vi "Translator.vi"(0 "Input":variant=variant("Function Name"=variant(string "Strip Path"), "Input Datatypes"=variant(string[] ["error", "int"]), "Inputs"=variant(string[] ["error in", "x"]), "Node refnum"=variant(refnum<vi> refnum), "Output Datatypes"=variant(string[] ["int"]), "Outputs"=variant(string[] ["a"])), 11 "error in (no error)":errorcluster) -> (4 "Output":variant=variant("Defines"=variant(string[] []), "Includes"=variant(string[] []), "Replaced Code"=variant(string "/* LabVIEW system function 'Strip Path' not found. */")), 15 "error out":errorcluster)   [LabVIEW 2014, in "LabVIEW Universal Trasncriptor Servo.lvlib"]
doc: "An example of how to create the Translator to convert the LabVIEW VIs to Arduino C code."
uses:
  LabVIEW Universal Trasncriptor Servo.lvlib
panel:
  out "Outputs":string[](array[string])
  out "Inputs":string[](array[string])
  out "Output Datatypes":string[](array[string])
  out "Input Datatypes":string[](array[string])
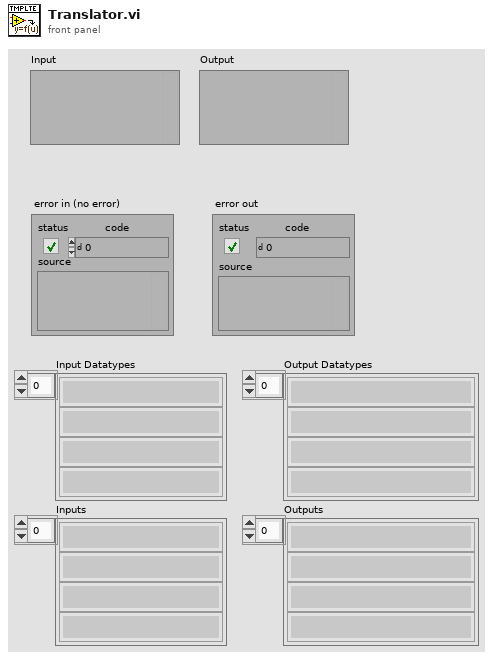
[diagram p1: front panel]
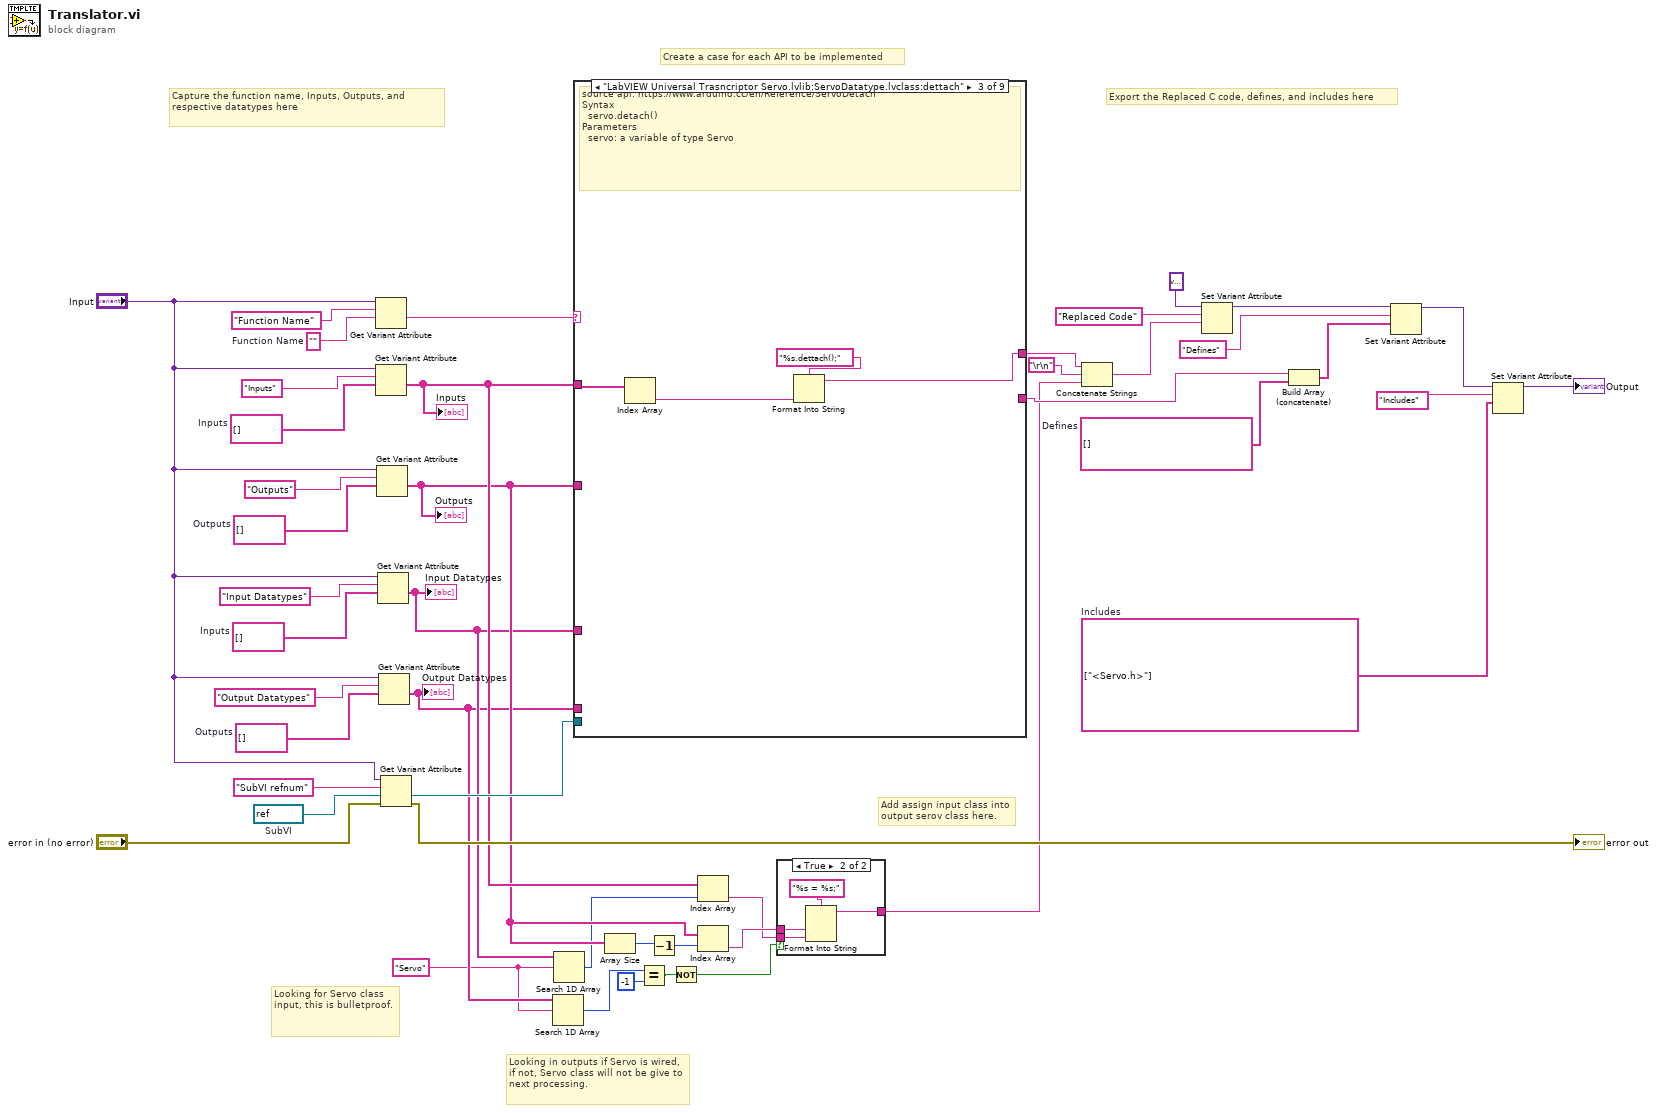
[diagram p0: block diagram]
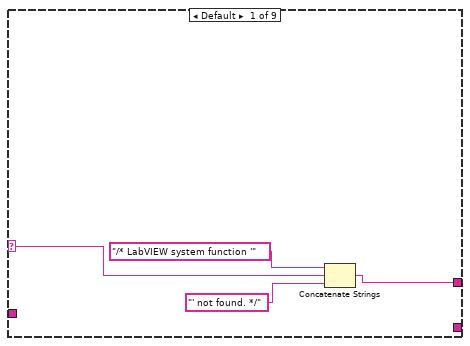
[diagram p3: hidden frame]
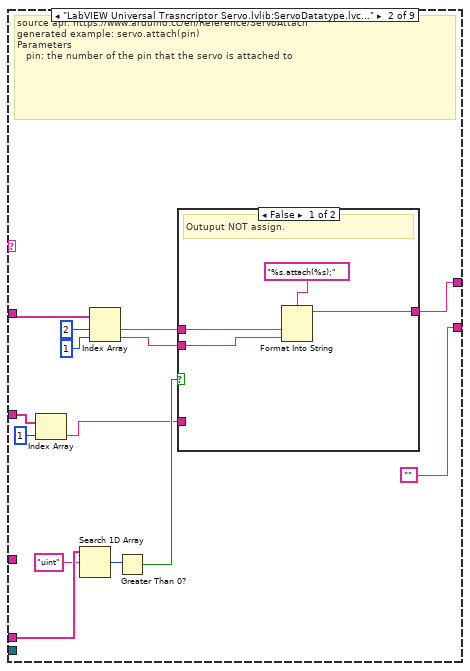
[diagram p4: hidden frame]
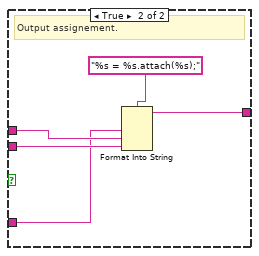
[diagram p5: hidden frame]
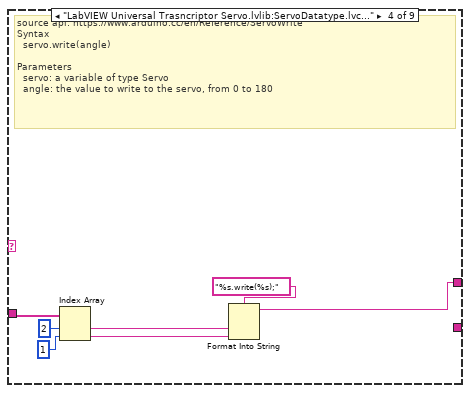
[diagram p6: hidden frame]
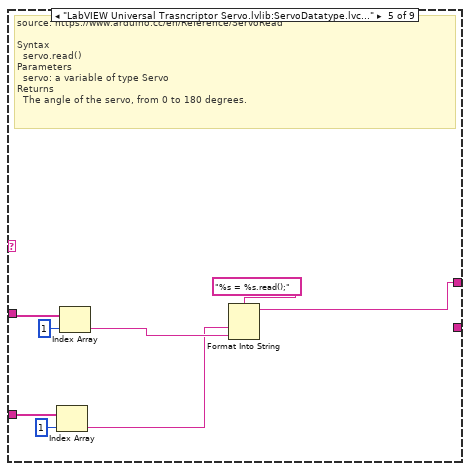
[diagram p7: hidden frame]
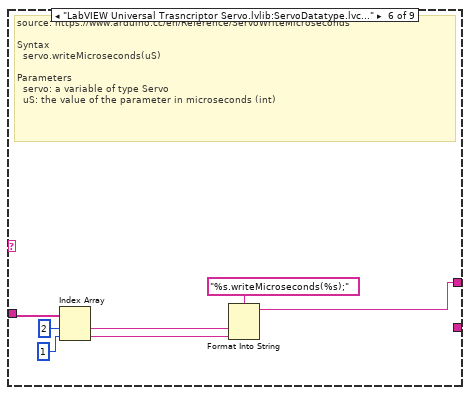
[diagram p8: hidden frame]
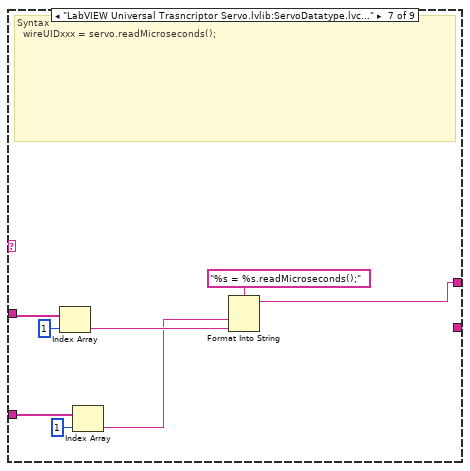
[diagram p9: hidden frame]
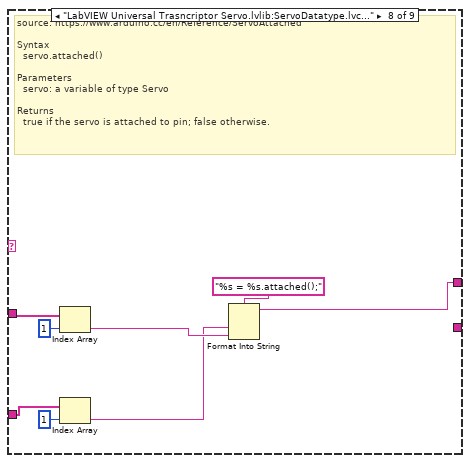
[diagram p10: hidden frame]
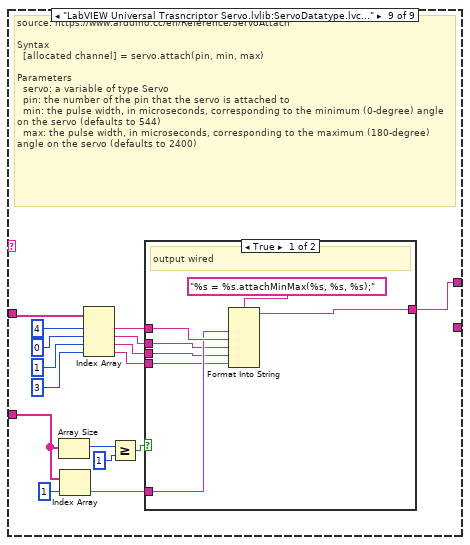
[diagram p11: hidden frame]
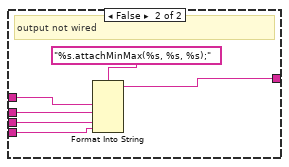
[diagram p12: hidden frame]
diagram:
  w2 = "Servo" ("format string")
  w26 = refnum<vi> refnum  # SubVI
  w21 = string[] []  # Defines
  w33 = string[] []  # Outputs
  w34 = string[] []  # Inputs
  w24 = string[] ["<Servo.h>"]  # Includes
  w42 = string[] []  # Outputs
  w43 = string[] []  # Inputs
  w44 = ""  # Function Name
  # "Looking for Servo class input, this is bulletproof."
  # "Looking in outputs if Servo is wired, if not, Servo class will not be give to next processing."
  # "Add assign input class into output serov class here."
  # "Capture the function name, Inputs, Outputs, and respective datatypes here"
  # "Export the Replaced C code, defines, and includes here"
  # "Create a case for each API to be implemented"
  n1 = Get Variant Attribute(Variant="Input", name="Function Name", default value (empty Variant)=w44) -> (value=w39:string)  [unwired: 1 in, 3 out]
  n2 = Get Variant Attribute(Variant="Input", name="Inputs", default value (empty Variant)=w43) -> (value=w10:string[])  [unwired: 1 in, 3 out]
  "Inputs" <- w10
  n3 = Get Variant Attribute(Variant="Input", name="Outputs", default value (empty Variant)=w42) -> (value=w9:string[])  [unwired: 1 in, 3 out]
  "Outputs" <- w9
  n4 = Get Variant Attribute(Variant="Input", name="Input Datatypes", default value (empty Variant)=w34) -> (value=w8:string[])  [unwired: 1 in, 3 out]
  "Input Datatypes" <- w8
  n5 = Get Variant Attribute(Variant="Input", name="Output Datatypes", default value (empty Variant)=w33) -> (value=w3:string[])  [unwired: 1 in, 3 out]
  "Output Datatypes" <- w3
  n6 = Get Variant Attribute(Variant="Input", name="SubVI refnum", default value (empty Variant)=w26, error in="error in (no error)") -> (value=w25:refnum<vi>, error out=→"error out":errorcluster)  [unwired: 2 out]
  n7 = Search 1D Array(1D array=w3, element=w2) -> (index of element=w1:i32)  [unwired: 1 in]
  n8 = Search 1D Array(1D array=w8, element=w2) -> (index of element=w6:i32)  [unwired: 1 in]
  n9 = case shown="\"LabVIEW Universal Trasncriptor Servo.lvlib:ServoDatatype.lvclass:dettach\"" w39 {
    selector: w39 -> [w49 _ _ _ _ _ _ _ _]
    tunnel: [w47 w62 w74 w81 w90 w97 w105 w113 w130] -> w14
    tunnel: w10 -> [_ w64 w76 w83 w91 w98 w106 w114 w131]
    tunnel: w9 -> [_ w57 _ _ w87 _ w101 w110 w125]
    tunnel: w8 -> [_ _ _ _ _ _ _ _ _]
    tunnel: w25 -> [_ _ _ _ _ _ _ _ _]
    tunnel: w3 -> [_ w56 _ _ _ _ _ _ _]
    tunnel: [_ "" _ _ _ _ _ _ _] -> w19
    frame Default {
      n10 = Concatenate Strings("/* LabVIEW system function '", w49, "' not found. */") -> (w47:string)
    }
    frame "LabVIEW Universal Trasncriptor Servo.lvlib:ServoDatatype.lvclass:attach" {
      # "source api: https://www.arduino.cc/en/Reference/ServoAttach\ngenerated example: servo.attach(pin)\nParameters\n   pin: the number of the pin that the servo is attached to"
      n11 = Index Array(array=w57, index=1) -> (element=w52:string)
      n12 = Search 1D Array(1D array=w56, element="uint") -> (index of element=w54:i32)  [unwired: 1 in]
      n13 = Index Array(array=w64, index #1=2 ("index"), index #2=1 ("index")) -> (element #1=w61:string, element #2=w59:string)
      n14 = Greater Than 0?(x=w54) -> (x > 0?=w53:bool)
      n15 = case shown="False" w53 {
        tunnel: [w67 w72] -> w62
        tunnel: w61 -> [w65 w70]
        tunnel: w59 -> [w66 w71]
        tunnel: w52 -> [_ w69]
        frame False {
          # "Outuput NOT assign."
          n16 = Format Into String(format string="%s.attach(%s);", w65, w66) -> (resulting string=w67:string)  [unwired: 2 in, 1 out]
        }
        frame True {
          # "Output assignement."
          n17 = Format Into String(format string="%s = %s.attach(%s);", w69, w70, w71) -> (resulting string=w72:string)  [unwired: 2 in, 1 out]
        }
      }
    }
    frame "LabVIEW Universal Trasncriptor Servo.lvlib:ServoDatatype.lvclass:dettach" {
      # "source api: https://www.arduino.cc/en/Reference/ServoDetach\nSyntax\n  servo.detach()\nParameters\n  servo: a variable of type Servo"
      n18 = Index Array(array=w76) -> (element=w75:string)  [unwired: 1 in]
      n19 = Format Into String(format string="%s.dettach();", w75) -> (resulting string=w74:string)  [unwired: 2 in, 1 out]
    }
    frame "LabVIEW Universal Trasncriptor Servo.lvlib:ServoDatatype.lvclass:write" {
      # "source api: https://www.arduino.cc/en/Reference/ServoWrite\nSyntax\n  servo.write(angle)\n\nParameters\n  servo: a variable of type Servo\n  angle: the value to write to the servo, from 0 to 180"
      n20 = Index Array(array=w83, index #1=2 ("index"), index #2=1 ("index")) -> (element #1=w82:string, element #2=w79:string)
      n21 = Format Into String(format string="%s.write(%s);", w82, w79) -> (resulting string=w81:string)  [unwired: 2 in, 1 out]
    }
    frame "LabVIEW Universal Trasncriptor Servo.lvlib:ServoDatatype.lvclass:read" {
      # "source: https://www.arduino.cc/en/Reference/ServoRead\n\nSyntax\n  servo.read()\nParameters\n  servo: a variable of type Servo\nReturns\n  The angle of the servo, from 0 to 180 degrees."
      n22 = Index Array(array=w87, index=1) -> (element=w85:string)
      n23 = Index Array(array=w91, index=1) -> (element=w86:string)
      n24 = Format Into String(format string="%s = %s.read();", w85, w86) -> (resulting string=w90:string)  [unwired: 2 in, 1 out]
    }
    frame "LabVIEW Universal Trasncriptor Servo.lvlib:ServoDatatype.lvclass:writeMicroseconds" {
      # "source: https://www.arduino.cc/en/Reference/ServoWriteMicroseconds \n\nSyntax\n  servo.writeMicroseconds(uS)\n\nParameters\n  servo: a variable of type Servo\n  uS: the value of the parameter in microseconds (int)"
      n25 = Index Array(array=w98, index #1=2 ("index"), index #2=1 ("index")) -> (element #1=w94:string, element #2=w93:string)
      n26 = Format Into String(format string="%s.writeMicroseconds(%s);", w94, w93) -> (resulting string=w97:string)  [unwired: 2 in, 1 out]
    }
    frame "LabVIEW Universal Trasncriptor Servo.lvlib:ServoDatatype.lvclass:readMicroseconds" {
      # "Syntax\n  wireUIDxxx = servo.readMicroseconds();"
      n27 = Index Array(array=w106, index=1) -> (element=w103:string)
      n28 = Index Array(array=w101, index=1) -> (element=w100:string)
      n29 = Format Into String(format string="%s = %s.readMicroseconds();", w100, w103) -> (resulting string=w105:string)  [unwired: 2 in, 1 out]
    }
    frame "LabVIEW Universal Trasncriptor Servo.lvlib:ServoDatatype.lvclass:attached" {
      # "source: https://www.arduino.cc/en/Reference/ServoAttached\n\nSyntax\n  servo.attached()\n\nParameters\n  servo: a variable of type Servo\n\nReturns\n  true if the servo is attached to pin; false otherwise."
      n30 = Index Array(array=w114, index=1) -> (element=w109:string)
      n31 = Index Array(array=w110, index=1) -> (element=w108:string)
      n32 = Format Into String(format string="%s = %s.attached();", w108, w109) -> (resulting string=w113:string)  [unwired: 2 in, 1 out]
    }
    frame "LabVIEW Universal Trasncriptor Servo.lvlib:ServoDatatype.lvclass:attachMinMax" {
      # "source: https://www.arduino.cc/en/Reference/ServoAttach\n\nSyntax\n  [allocated channel] = servo.attach(pin, min, max)\n\nParameters\n  servo: a variable of type Servo\n  pin: the number of the pin that the servo is attached to\n  min: the pulse width, in microseconds, corresponding to the minimum (0-degree) angle on the servo (defaults to 544)\n  max: the pulse width, in microseconds, corresponding to the maximum (180-degree) angle on the servo (defaults to 2400)"
      n33 = Array Size(array=w125) -> (size(s)=w123:i32)
      n34 = Index Array(array=w125, index=1) -> (element=w126:string)
      n35 = Index Array(array=w131, index #1=4 ("index"), index #2=0 ("index"), index #3=1 ("index"), index #4=3 ("index")) -> (element #1=w127:string, element #2=w118:string, element #3=w117:string, element #4=w116:string)
      n36 = Greater Or Equal?(x=w123, y=1) -> (x >= y?=w124:bool)
      n37 = case shown="True" w124 {
        tunnel: [w137 w143] -> w130
        tunnel: w127 -> [w136 w142]
        tunnel: w126 -> [w135 _]
        tunnel: w118 -> [w134 w141]
        tunnel: w117 -> [w133 w140]
        tunnel: w116 -> [w132 w139]
        frame True {
          # "output wired"
          n38 = Format Into String(format string="%s = %s.attachMinMax(%s, %s, %s);", w135, w136, w134, w133, w132) -> (resulting string=w137:string)  [unwired: 2 in, 1 out]
        }
        frame False {
          # "output not wired"
          n39 = Format Into String(format string="%s.attachMinMax(%s, %s, %s);", w142, w141, w140, w139) -> (resulting string=w143:string)  [unwired: 2 in, 1 out]
        }
      }
    }
  }
  n40 = Array Size(array=w9) -> (size(s)=w18:i32)
  n41 = Equal?(x=w1, y=-1 ("index of element")) -> (x = y?=w5:bool)
  n42 = Decrement(x=w18) -> (x-1=w17:i32)
  n43 = Not(x=w5) -> (.not. x?=w4:bool)
  n44 = Index Array(array=w10, index=w6) -> (element=w15:string)
  n45 = Index Array(array=w9, index=w17) -> (element=w16:string)
  n46 = case shown="True" w4 {
    tunnel: w16 -> [_ w147]
    tunnel: w15 -> [_ w146]
    tunnel: [_ w145] -> w11
    frame False {
    }
    frame True {
      n47 = Format Into String(format string="%s = %s;", w147, w146) -> (resulting string=w145:string)  [unwired: 2 in, 1 out]
    }
  }
  n48 = Concatenate Strings(w14, "\r\n", w11) -> (w13:string)
  n49 = Set Variant Attribute(Variant=variant ("variant"), name="Replaced Code", value=w13) -> (Variant out=w31:variant)  [unwired: 1 in, 2 out]
  n50 = Build Array (concatenate)(w19, w21) -> (w20:string[])
  n51 = Set Variant Attribute(Variant=w31, name="Defines", value=w20) -> (Variant out=w30:variant)  [unwired: 1 in, 2 out]
  n52 = Set Variant Attribute(Variant=w30, name="Includes", value=w24) -> (Variant out=→"Output":variant)  [unwired: 1 in, 2 out]
